vi "Generate Description String.vi"(8 "error in (no error)":errorcluster, 11 "heater_parent in":refnum<class "heater_parent.lvclass">) -> (0 "error out":errorcluster, 2 "Description String":string, 3 "heater_parent out":refnum<class "heater_parent.lvclass">)   [LabVIEW 2020, in "polar_bear_plus_drivers.lvlib" / "heater_parent.lvclass"]
doc: "Generate a string describing the instrument resource. This string can be loaded later with the \"Parse Description String\" VI to connect to the instrument again."
uses:
  <instrlib>/RxnRover/Driver Polar Bear Plus/heater_parent/heater_parent.lvclass
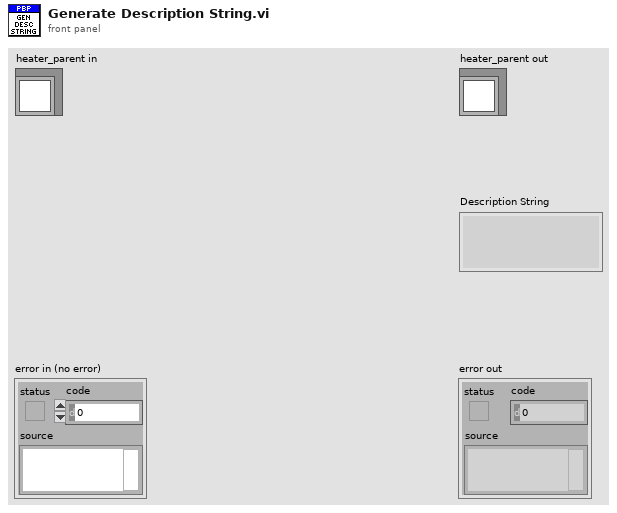
[diagram p1: front panel]
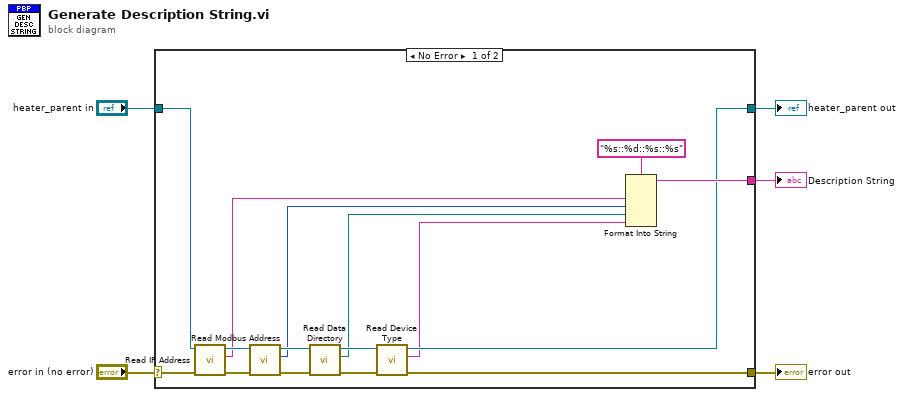
[diagram p0: block diagram]
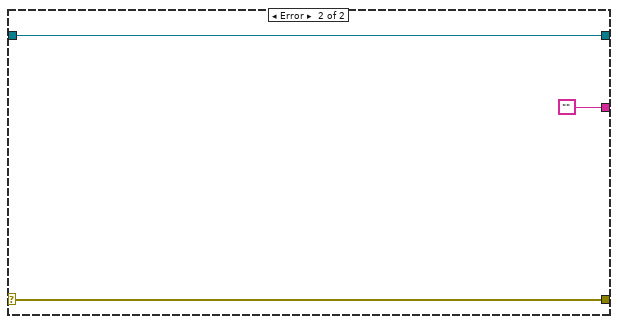
[diagram p2: hidden frame]
diagram:
  n1 = case shown="No Error" "error in (no error)" {
    selector: "error in (no error)" -> [w21 w24]
    tunnel: [w7 w24] -> w4
    tunnel: [w9 w23] -> w2
    tunnel: "heater_parent in" -> [w16 w23]
    tunnel: [w10 ""] -> w1
    frame No Error {
      n2 = call-dynamic "Read IP Address.vi"("error in (no error)"=w21, "heater_parent in"=w16) -> ("error out"=w20:errorcluster, "IP Address"=w13:string, "heater_parent out"=w18:refnum<class "heater_parent.lvclass">)  [unwired: 7 in]
      n3 = call-dynamic "Read Modbus Address.vi"("error in (no error)"=w20, "heater_parent in"=w18) -> ("error out"=w19:errorcluster, "Modbus Address"=w12:u8, "heater_parent out"=w17:refnum<class "heater_parent.lvclass">)  [unwired: 7 in]
      n4 = call-dynamic "Read Data Directory.vi"("error in (no error)"=w19, "heater_parent in"=w17) -> ("error out"=w8:errorcluster, "Data Directory"=w11:path, "heater_parent out"=w15:refnum<class "heater_parent.lvclass">)  [unwired: 7 in]
      n5 = call-dynamic "Read Device Type.vi"("error in (no error)"=w8, "heater_parent in"=w15) -> ("error out"=w7:errorcluster, "Device Type"=w6:string, "heater_parent out"=w9:refnum<class "heater_parent.lvclass">)  [unwired: 7 in]
      n6 = Format Into String(format string="%s::%d::%s::%s", w13, w12, w11, w6) -> (resulting string=w10:string)  [unwired: 2 in, 1 out]
    }
    frame Error {
    }
  }
  "error out" <- w4
  "heater_parent out" <- w2
  "Description String" <- w1
